vi "render_zernikes.vi"(0 "Size":i32=50, 1 "Coefficients":dbl[](array[slide]) scale=-5.0..5.0) -> (5 "Phase Map":dbl[][](array[numeric]))   [LabVIEW 2019]
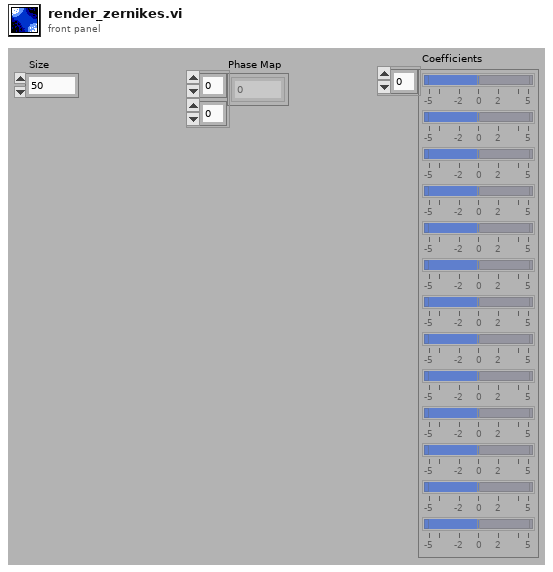
[diagram p1: front panel]
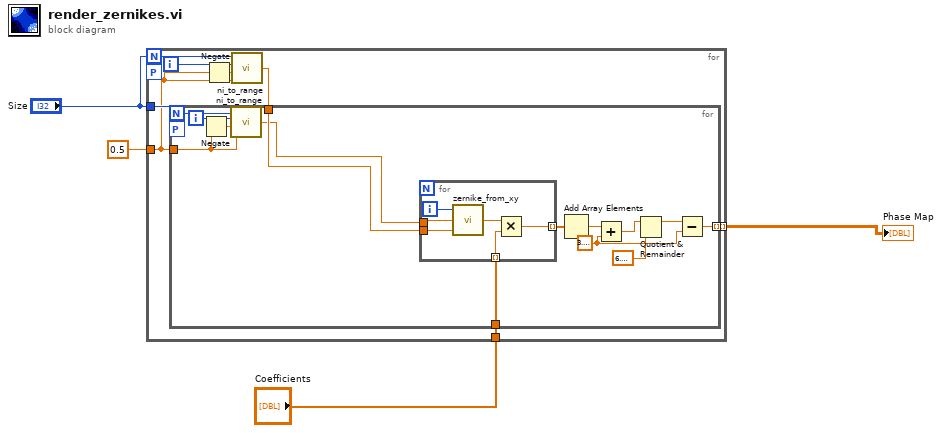
[diagram p0: block diagram]
diagram:
  n1 = for {
    N: "Size" -> [w11]
    tunnel: "Size" -> [w12]
    tunnel: 0.5 ("end") -> [w5]
    tunnel: "Coefficients" -> [w7]
    tunnel: [w6] -> w1 mode=indexing
    workers-P: _ -> [_]
    i -> [w10]
    n2 = Negate(x=w5) -> (-x=w8:dbl)
    n3 = call "ni_to_range.vi"("end"=w5, "start"=w8, "i"=w10, "N"=w11) -> ("current value (runs from start to end in N steps)"=w9:dbl)
    n4 = for {
      N: w12 -> [w26]
      tunnel: w9 -> [w22]
      tunnel: w5 -> [w23]
      tunnel: w7 -> [w20]
      tunnel: [w17] -> w6 mode=indexing
      workers-P: _ -> [_]
      i -> [w25]
      w14 = 3.141592653589793
      n5 = Negate(x=w23) -> (-x=w24:dbl)
      n6 = call "ni_to_range.vi"("end"=w23, "start"=w24, "i"=w25, "N"=w26) -> ("current value (runs from start to end in N steps)"=w21:dbl)
      n7 = for {
        tunnel: w21 -> [w32]
        tunnel: w22 -> [w31]
        tunnel: w20 -> [w28] mode=indexing
        tunnel: [w27] -> w19 mode=indexing
        i -> [w30]
        n8 = call "zernike_from_xy.vi"("y (-.5 to .5)"=w31, "x (-.5 to .5)"=w32, "Numeric"=w30) -> ("z"=w29:dbl)
        n9 = Multiply(x=w29, y=w28) -> (x*y=w27:dbl)
      }
      n10 = Add Array Elements(numeric array=w19) -> (sum=w18:dbl)
      n11 = Add(x=w18, y=w14) -> (x+y=w15:dbl)
      n12 = Quotient & Remainder(x=w15, y=6.283185307179586) -> (x-y*floor(x/y)=w16:dbl)  [unwired: 1 out]
      n13 = Subtract(x=w16, y=w14) -> (x-y=w17:dbl)
    }
  }
  "Phase Map" <- w1
